vi "Get_Sub_Collection.vi"(8 "error in (no error)":errorcluster caption="entrée d'erreur (pas d'erreur)", 11 "Firebase Benches en entrée":refnum<class "Firebase Benches_Booleen.lvclass">) -> (0 "error out":errorcluster caption="sortie d'erreur", 3 "Firebase Benches en sortie":refnum<class "Firebase Benches_Booleen.lvclass">)   [LabVIEW 2020, in "Library Instrument & Equipement.lvlib" / "Library FireBase.lvlib" / "Firebase Benches_Booleen.lvclass"]
doc: "Return the documents present in the test collection for each DATA read with Get_Data\nPlease initialise the following values\n - Name BDD\n - Document of test sequence\n - API Key\n - Nb To Read"
uses:
  Firebase Benches_Booleen.lvclass
  C:/Users/ngarcin/OneDrive - Altyor/Standard TB/Class/Firebase/Source/Firebase PCBA/Firebase Benches.lvclass
  C:/Users/ngarcin/OneDrive - Altyor/Standard TB/Class/Firebase/Source/Firebase Driver/Firebase Driver.lvclass
  Firebase Benches_Booleen.lvclass/Firebase Benches_Booleen.ctl
  JSON API/JSON Value/Set from JSON string.vi
  JSON API/JSON Value/JSON Value.lvclass
  Firebase Benches.lvclass
  JSON API/Variant JSON/Variant JSON.lvlib
  JSON API/Get Polymorphic/JSON GetSet.lvlib
  Firebase Driver/Firebase Driver.lvclass
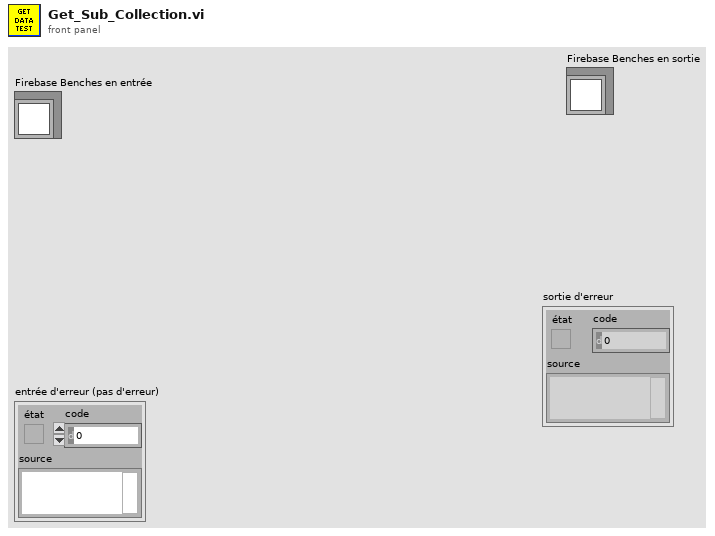
[diagram p1: front panel]
types:
  T1 = cluster{"name":string, "fields":cluster{"Result":cluster{"booleanValue":bool}, "Name":cluster{"stringValue":string}, "StartOfTest":cluster{"timestampValue":string}, "EndOfTest":cluster{"timestampValue":string}, "limit":cluster{"mapValue":cluster{"fields":cluster{"Lower":cluster{"stringValue":string}, "Upper":cluster{"stringValue":string}}}}, "Value":cluster{"booleanValue":bool}, "Type":cluster{"stringValue":string}, "MainTest":cluster{"stringValue":string}}}[][]
  T2 = cluster{"name":string, "fields":cluster{"Result":cluster{"booleanValue":bool}, "CreationDate":cluster{"timestampValue":string}, "Batch":cluster{"stringValue":string}, "SerialNumber":cluster{"stringValue":string}, "EndOfProduction":cluster{"timestampValue":string}, "FW_Version":cluster{"mapValue":cluster{"fields":cluster{"Bootloader":cluster{"mapValue":cluster{"fields":cluster{"File_Name":cluster{"stringValue":string}, "Version":cluster{"mapValue":cluster{"fields":cluster{"Major":cluster{"stringValue":string}, "Minor":cluster{"stringValue":string}}}}, "Checksum":cluster{"stringValue":string}}}}, "SoftDevice":cluster{"mapValue":cluster{"fields":cluster{"File_Name":cluster{"stringValue":string}, "Version":cluster{"mapValue":cluster{"fields":cluster{"Major":cluster{"stringValue":string}, "Minor":cluster{"stringValue":string}}}}, "Checksum":cluster{"stringValue":string}}}}, "DFU":cluster{"mapValue":cluster{"fields":cluster{"File_Name":cluster{"stringValue":string}, "Version":cluster{"mapValue":cluster{"fields":cluster{"Major":cluster{"stringValue":string}, "Minor":cluster{"stringValue":string}}}}, "Checksum":cluster{"stringValue":string}}}}}}}, "PartNumber":cluster{"stringValue":string}, "OrderNumber":cluster{"stringValue":string}, "Operator":cluster{"stringValue":string}}}[]
  T3 = cluster{"name":string, "fields":cluster{"Result":cluster{"booleanValue":bool}, "Name":cluster{"stringValue":string}, "StartOfTest":cluster{"timestampValue":string}, "EndOfTest":cluster{"timestampValue":string}, "limit":cluster{"mapValue":cluster{"fields":cluster{"Lower":cluster{"stringValue":string}, "Upper":cluster{"stringValue":string}}}}, "Value":cluster{"booleanValue":bool}, "Type":cluster{"stringValue":string}, "MainTest":cluster{"stringValue":string}}}[]
  T4 = cluster{"documents":cluster{"name":string, "fields":cluster{"Result":cluster{"booleanValue":bool}, "Name":cluster{"stringValue":string}, "StartOfTest":cluster{"timestampValue":string}, "EndOfTest":cluster{"timestampValue":string}, "limit":cluster{"mapValue":cluster{"fields":cluster{"Lower":cluster{"stringValue":string}, "Upper":cluster{"stringValue":string}}}}, "Value":cluster{"booleanValue":bool}, "Type":cluster{"stringValue":string}, "MainTest":cluster{"stringValue":string}}}[], "nextPageToken":string}
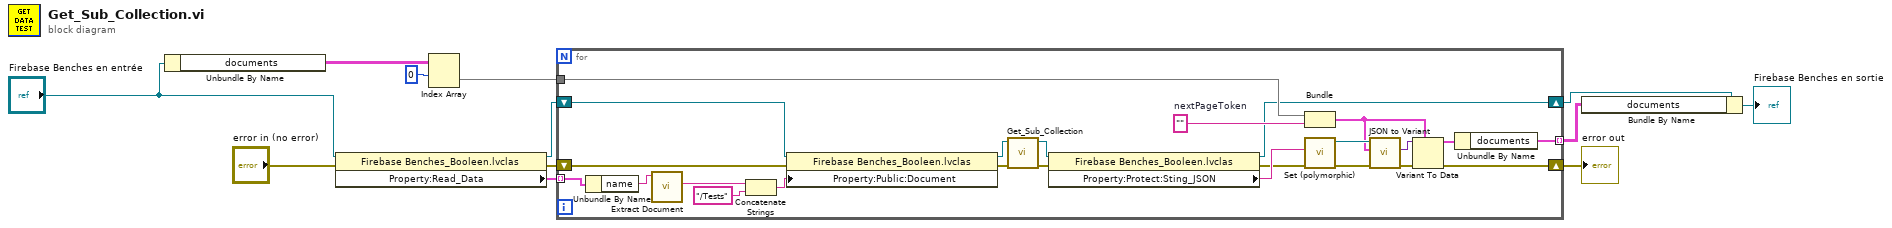
[diagram p0: block diagram]
diagram:
  n1 = Unbundle By Name("Firebase Benches en entrée") -> ("documents"=w9:T1)
  n2 = property class="Firebase Benches_Booleen.lvclas"(reference="Firebase Benches en entrée", error in="error in (no error)") -> (reference out=w4:refnum<class "Firebase Benches_Booleen.lvclass">, error out=w2:errorcluster, "Property:Read_Data"=w1:T2)
  n3 = Index Array(array=w9, index (row)=0 ("indice (ligne)")) -> (element=w8:T3)  [unwired: 1 in]
  n4 = for {
    tunnel: [w29] -> w11 mode=indexing
    shift-right: [w13] -> w6
    shift-left: w4 -> [w28]
    shift-right: [w14] -> w12
    shift-left: w2 -> [w27]
    tunnel: w1 -> [w26] mode=indexing
    tunnel: w8 -> [w17]
    w31 = ""  # nextPageToken
    n5 = Unbundle By Name(w26) -> ("name"=w25:string)
    n6 = call "Extract Document.vi"("Name"=w25) -> ("Source"=w24:string)  [unwired: 9 in, 1 out]
    n7 = Concatenate Strings(w24, "/Tests" ("chaîne")) -> (w22:string)
    n8 = property class="Firebase Benches_Booleen.lvclas"(reference=w28, error in=w27, "Property:Public:Document"=w22) -> (reference out=w18:refnum<class "Firebase Benches_Booleen.lvclass">, error out=w21:errorcluster)
    n9 = call-parent "Get_Sub_Collection.vi"("error in (no error)"=w21, "Firebase Benches en entrée"=w18) -> ("error out"=w20:errorcluster, "Firebase Benches en sortie"=w19:refnum<class "Firebase Benches_Booleen.lvclass">)  [unwired: 8 in]
    n10 = property class="Firebase Benches_Booleen.lvclas"(reference=w19, error in=w20) -> (reference out=w13:refnum<class "Firebase Benches_Booleen.lvclass">, error out=w16:errorcluster, "Property:Protect:Sting_JSON"=w33:string)
    n11 = Bundle("documents"=w17, "nextPageToken"=w31) -> (w30:T4)  [unwired: 1 in]
    n12 = call-poly "Set (polymorphic).vi"("error in (no error)"=w16, "JSON stream"=w33) -> ("error out"=w34:errorcluster, "JSON Value out"=w36:refnum<class "JSON Value.lvclass">)  [unwired: 7 in, 1 out]
    n13 = call "JSON to Variant.vi"("error in (no error)"=w34, "Variant (Data Type)"=w30, "JSON Value"=w36) -> ("error out"=w35:errorcluster, "Variant out"=w15:variant)  [unwired: 7 in]
    n14 = Variant To Data(error in=w35, type=w30, Variant=w15) -> (data=w32:T4, error out=w14:errorcluster)
    n15 = Unbundle By Name(w32) -> ("documents"=w29:T3)
  }
  "error out" <- w12
  n16 = Bundle By Name(cluster=w6, "documents"=w11) -> (→"Firebase Benches en sortie":refnum<class "Firebase Benches_Booleen.lvclass">)
